vi "Test Different Internal ImageResIDs.vi"(8 "error in (no error)":errorcluster) -> (0 "error out":errorcluster)   [LabVIEW 2026, in "VILab.lvlib"]
uses:
  VILab.lvlib
  SubVIs/Find Resource by Type (String).vi
  CTLs/Resource.ctl
  <vilib>/Utility/traverseref.llb/VI Scripting - Traverse.lvlib
  <vilib>/Utility/traverseref.llb/TRef TravTarget.ctl
panel:
  out "i":i32
  out "Last Error":errorcluster
  out "Working IDs":i32[](array[numeric])
  in  "stop":bool
  # "tried up to -5000"
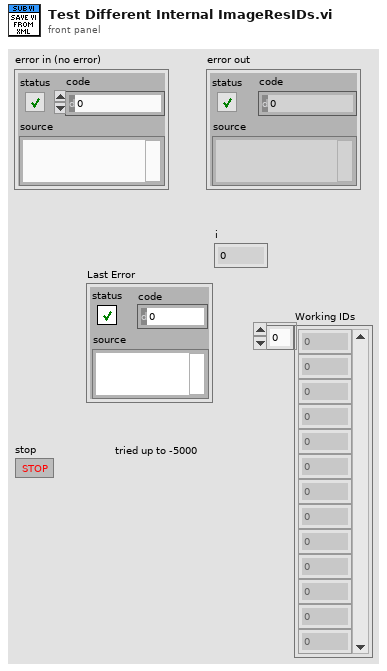
[diagram p1: front panel]
types:
  T1 = typedef "TRef TravTarget.ctl" = enum16{"FP", "BD", "Other"}
  T2 = typedef "VILab.lvlib/Resource.ctl" = cluster{"type":u32, "id":i32, "name":string, "binary data":string}
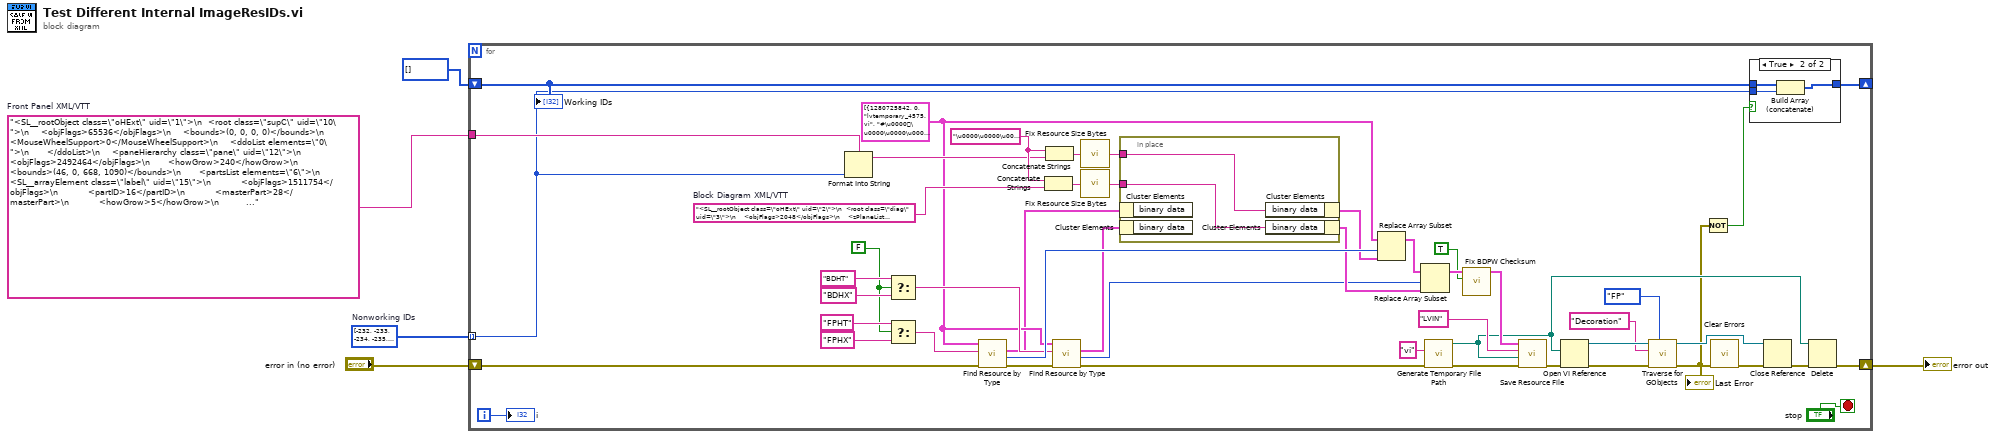
[diagram p0: block diagram]
diagram:
  w1 = i32[] [-232, -233, -234, -235, -236, -237, -367, -368, -369, -370, -371, -372, -392, -501, -502, -503, -504, -532, -542, -642, -643, -646, -647, -765, -770, -784, -785, -840, -841, -842, -843, -844, -845, -846, -847, -848, -849, -850, -851, -852, -853, -854, -855, -856, -857, -858, -859, -860, -861, -862, -863, -864, -865, -866, -867, -868, -869, -870, -871, -872, -873, -874, -875, -876, -877, -878, -879, -880, -881, -882, -883, -884, -885, -886, -887, -888, -889, -890, -891, -892, -893, -894, -895, -896, -897, -898, -899, -900, -901, -902, -903, -904, -905, -906, -907, -908, -909, -910, -911, -912, -913, -914, -915, -916, -917, -918, -919, -920, -921, -922, -923, -924, -925, -926, -927, -928, -929, -930, -931, -932, -933, -934, -935, -936, -937, -938, -939, -940, -941, -942, -943, -944, -945, -946, -947, -948, -949, -950, -951, -952, -953, -954, -955, -956, -957, -958, -959, -960, -961, -962, -963, -964, -965, -966, -967, -968, -969, -970, -971, -972, -973, -974, -975, -976, -977, -978, -979, -980, -981, -982, -983, -984, -985, -986, -987, -988, -989, -990, -991, -992, -993, -994, -995, -996, -997, -998, -999, -1031, -1032, -1033, -1034, -1035, -1036, -1037, -1038, -1039, -1040, -1041, -1042, -1043, -1044, -1045, -1046, -1047, -1048, -1049, -1050, -1051, -1052, -1053, -1054, -1055, -1056, -1057, -1058, -1059, -1060, -1061, -1062, -1063, -1064, -1065, -1066, -1067, -1068, -1069, -1070, -1071, -1072, -1073, -1074, -1075, -1076, -1077, -1078, -1079, -1080, -1081, -1082, -1083, -1084, -1085, -1086, -1087, -1088, -1089, -1090, -1091, -1092, -1093, -1094, -1095, -1096, -1097, -1098, -1099, -1100, -1101, -1102, -1103, -1104, -1105, -1106, -1107, -1108, -1109, -1110, -1111, -1112, -1113, -1114, -1115, -1116, -1117, -1118, -1119, -1120, -1121, -1122, -1123, -1124, -1125, -1126, -1127, -1128, -1129, -1130, -1131, -1132, -1133, -1134, -1135, -1136, -1137, -1138, -1139, -1140, -1141, -1142, -1143, -1144, -1145, -1146, -1147, -1148, -1149, -1150, -1151, -1152, -1153, -1154, -1155, -1156, -1157, -1158, -1159, -1160, -1161, -1162, -1163, -1164, -1165, -1166, -1167, -1168, -1169, -1170, -1171, -1172, -1173, -1174, -1175, -1176, -1177, -1178, -1179, -1180, -1181, -1182, -1183, -1184, -1185, -1186, -1187, -1188, -1189, -1190, -1191, -1192, -1193, -1194, -1195, -1196, -1197, -1198, -1199, -1200, -1201, -1202, -1203, -1204, -1205, -1206, -1207, -1208, -1209, -1210, -1211, -1212, -1213, -1214, -1215, -1216, -1217, -1218, -1219, -1220, -1221, -1222, -1223, -1224, -1225, -1226, -1227, -1228, -1229, -1230, -1231, -1232, -1233, -1234, -1235, -1236, -1237, -1238, -1239, -1240, -1241, -1242, -1243, -1244, -1245, -1246, -1247, -1248, -1249, -1250, -1251, -1252, -1253, -1254, -1255, -1256, -1257, -1258, -1259, -1260, -1261, -1262, -1263, -1264, -1265, -1266, -1267, -1268, -1269, -1270, -1271, -1272, -1273, -1274, -1275, -1276, -1277, -1278, -1279, -1280, -1281, -1282, -1283, -1284, -1285, -1286, -1287, -1288, -1289, -1290, -1291, -1292, -1293, -1294, -1295, -1296, -1297, -1298, -1299, -1300, -1301, -1302, -1303, -1304, -1305, -1306, -1307, -1308, -1309, -1310, -1311, -1312, -1313, -1314, -1315, -1316, -1317, -1318, -1319, -1320, -1321, -1322, -1323, -1324, -1325, -1326, -1327, -1328, -1329, -1330, -1331, -1332, -1333, -1334, -1335, -1336, -1337, -1338, -1339, -1340, -1341, -1342, -1343, -1344, -1345, -1346, -1347, -1348, -1349, -1350, -1351, -1352, -1353, -1354, -1355, -1356, -1357, -1358, -1359, -1360, -1361, -1362, -1363, -1364, -1365, -1366, -1367, -1368, -1369, -1370, -1371, -1372, -1373, -1374, -1375, -1376, -1377, -1378, -1379, -1380, -1381, -1382, -1383, -1384, -1385, -1386, -1387, -1388, -1389, -1390, -1391, -1392, -1393, -1394, -1395, -1396, -1397, -1398, -1399, -1400, -1401, -1402, -1403, -1404, -1405, -1406, -1407, -1408, -1409, -1410, -1411, -1412, -1413, -1414, -1415, -1416, -1417, -1418, -1419, -1420, -1421, -1422, -1423, -1424, -1425, -1426, -1427, -1428, -1429, -1430, -1431, -1432, -1433, -1434, -1435, -1436, -1437, -1438, -1439, -1440, -1441, -1442, -1443, -1444, -1445, -1446, -1447, -1448, -1449, -1450, -1451, -1452, -1453, -1454, -1455, -1456, -1457, -1458, -1459, -1460, -1461, -1462, -1463, -1464, -1465, -1466, -1467, -1468, -1469, -1470, -1471, -1472, -1473, -1474, -1475, -1476, -1477, -1478, -1479, -1480, -1481, -1482, -1483, -1484, -1485, -1486, -1487, -1488, -1489, -1490, -1491, -1492, -1493, -1494, -1495, -1496, -1497, -1498, -1499, -1500, -1501, -1502, -1503, -1504, -1505, -1506, -1507, -1508, -1509, -1510, -1511, -1512, -1513, -1514, -1515, -1516, -1517, -1518, -1519, -1520, -1521, -1522, -1523, -1524, -1525, -1526, -1527, -1528, -1529, -1530, -1531, -1532, -1533, -1534, -1535, -1536, -1537, -1538, -1539, -1540, -1541, -1542, -1543, -1544, -1545, -1546, -1547, -1548, -1549, -1550, -1551, -1552, -1553, -1554, -1555, -1556, -1557, -1558, -1559, -1560, -1561, -1562, -1563, -1564, -1565, -1566, -1567, -1568, -1569, -1570, -1571, -1572, -1573, -1574, -1575, -1576, -1577, -1578, -1579, -1580, -1581, -1582, -1583, -1584, -1585, -1586, -1587, -1588, -1589, -1590, -1591, -1592, -1593, -1594, -1595, -1596, -1597, -1598, -1599, -1600, -1601, -1602, -1603, -1604, -1605, -1606, -1607, -1608, -1609, -1610, -1611, -1612, -1613, -1614, -1615, -1616, -1617, -1618, -1619, -1620, -1621, -1622, -1623, -1624, -1625, -1626, -1627, -1628, -1629, -1630, -1631, -1632, -1633, -1634, -1635, -1636, -1637, -1638, -1639, -1640, -1641, -1642, -1643, -1644, -1645, -1646, -1647, -1648, -1649, -1650, -1651, -1652, -1653, -1654, -1655, -1656, -1657, -1658, -1659, -1660, -1661, -1662, -1663, -1664, -1665, -1666, -1667, -1668, -1669, -1670, -1671, -1672, -1673, -1674, -1675, -1676, -1677, -1678, -1679, -1680, -1681, -1682, -1683, -1684, -1685, -1686, -1687, -1688, -1689, -1690, -1691, -1692, -1693, -1694, -1695, -1696, -1697, -1698, -1699, -1700, -1701, -1702, -1703, -1704, -1705, -1706, -1707, -1708, -1709, -1710, -1711, -1712, -1713, -1714, -1715, -1716, -1717, -1718, -1719, -1720, -1721, -1722, -1723, -1724, -1725, -1726, -1727, -1728, -1729, -1730, -1731, -1732, -1733, -1734, -1735, -1736, -1737, -1738, -1739, -1740, -1741, -1742, -1743, -1744, -1745, -1746, -1747, -1748, -1749, -1750, -1751, -1752, -1753, -1754, -1755, -1756, -1757, -1758, -1759, -1760, -1761, -1762, -1763, -1764, -1765, -1766, -1767, -1768, -1769, -1770, -1771, -1772, -1773, -1774, -1775, -1776, -1777, -1778, -1779, -1780, -1781, -1782, -1783, -1784, -1785, -1786, -1787, -1788, -1789, -1790, -1791, -1792, -1793, -1794, -1795, -1796, -1797, -1798, -1799, -1800, -1801, -1802, -1803, -1804, -1805, -1806, -1807, -1808, -1809, -1810, -1811, -1812, -1813, -1814, -1815, -1816, -1817, -1818, -1819, -1820, -1821, -1822, -1823, -1824, -1825, -1826, -1827, -1828, -1829, -1830, -1831, -1832, -1833, -1834, -1835, -1836, -1837, -1838, -1839, -1840, -1841, -1842, -1843, -1844, -1845, -1846, -1847, -1848, -1849, -1850, -1851, -1852, -1853, -1854, -1855, -1856, -1857, -1858, -1859, -1860, -1861, -1862, -1863, -1864, -1865, -1866, -1867, -1868, -1869, -1870, -1871, -1872, -1873, -1874, -1875, -1876, -1877, -1878, -1879, -1880, -1881, -1882, -1883, -1884, -1885, -1886, -1887, -1888, -1889, -1890, -1891, -1892, -1893, -1894, -1895, -1896, -1897, -1898, -1899, -1900, -1901, -1902, -1903, -1904, -1905, -1906, -1907, -1908, -1909, -1910, -1911, -1912, -1913, -1914, -1915, -1916, -1917, -1918, -1919, -1920, -1921, -1922, -1923, -1924, -1925, -1926, -1927, -1928, -1929, -1930, -1931, -1932, -1933, -1934, -1935, -1936, -1937, -1938, -1939, -1940, -1941, -1942, -1943, -1944, -1945, -1946, -1947, -1948, -1949, -1950, -1951, -1952, -1953, -1954, -1955, -1956, -1957, -1958, -1959, -1960, -1961, -1962, -1963, -1964, -1965, -1966, -1967, -1968, -1969, -1970, -1971, -1972, -1973, -1974, -1975, -1976, -1977, -1978, -1979, -1980, -1981, -1982, -1983, -1984, -1985, -1986, -1987, -1988, -1989, -1990, -1991, -1992, -1993, -1994, -1995, -1996, -1997, -1998, -1999, -2110, -2111, -2112, -2113, -2114, -2115, -2116, -2117, -2118, -2119, -2120, -2121, -2122, -2123, -2124, -2125, -2126, -2127, -2128, -2129, -2130, -2131, -2132, -2133, -2134, -2135, -2136, -2137, -2138, -2139, -2140, -2141, -2142, -2143, -2144, -2145, -2146, -2147, -2148, -2149, -2150, -2151, -2152, -2153, -2154, -2155, -2156, -2157, -2158, -2159, -2160, -2161, -2162, -2163, -2164, -2165, -2166, -2167, -2168, -2169, -2170, -2171, -2172, -2173, -2174, -2175, -2176, -2177, -2178, -2179, -2180, -2181, -2182, -2183, -2184, -2185, -2186, -2187, -2188, -2189, -2190, -2191, -2192, -2193, -2194, -2195, -2196, -2197, -2198, -2199, -2200, -2201, -2202, -2203, -2204, -2205, -2206, -2207, -2208, -2209, -2210, -2211, -2212, -2213, -2214, -2215, -2216, -2217, -2218, -2219, -2220, -2221, -2222, -2223, -2224, -2225, -2226, -2227, -2228, -2229, -2230, -2231, -2232, -2233, -2234, -2235, -2236, -2237, -2238, -2239, -2240, -2241, -2242, -2243, -2244, -2245, -2246, -2247, -2248, -2249, -2250, -2251, -2252, -2253, -2254, -2255, -2256, -2257, -2258, -2259, -2260, -2261, -2262, -2263, -2264, -2265, -2266, -2267, -2268, -2269, -2270, -2271, -2272, -2273, -2274, -2275, -2276, -2277, -2278, -2279, -2280, -2281, -2282, -2283, -2284, -2285, -2286, -2287, -2288, -2289, -2290, -2291, -2292, -2293, -2294, -2295, -2296, -2297, -2298, -2299, -2300, -2301, -2302, -2303, -2304, -2305, -2306, -2307, -2308, -2309, -2310, -2311, -2312, -2313, -2314, -2315, -2316, -2317, -2318, -2319, -2320, -2321, -2322, -2323, -2324, -2325, -2326, -2327, -2328, -2329, -2330, -2331, -2332, -2333, -2334, -2335, -2336, -2337, -2338, -2339, -2340, -2341, -2342, -2343, -2344, -2345, -2346, -2347, -2348, -2349, -2350, -2351, -2352, -2353, -2354, -2355, -2356, -2357, -2358, -2359, -2360, -2361, -2362, -2363, -2364, -2365, -2366, -2367, -2368, -2369, -2370, -2371, -2372, -2373, -2374, -2375, -2376, -2377, -2378, -2379, -2380, -2381, -2382, -2383, -2384, -2385, -2386, -2387, -2388, -2389, -2390, -2391, -2392, -2393, -2394, -2395, -2396, -2397, -2398, -2399, -2400, -2401, -2402, -2403, -2404, -2405, -2406, -2407, -2408, -2409, -2410, -2411, -2412, -2413, -2414, -2415, -2416, -2417, -2418, -2419, -2420, -2421, -2422, -2423, -2424, -2425, -2426, -2427, -2428, -2429, -2430, -2431, -2432, -2433, -2434, -2435, -2436, -2437, -2438, -2439, -2440, -2441, -2442, -2443, -2444, -2445, -2446, -2447, -2448, -2449, -2450, -2451, -2452, -2453, -2454, -2455, -2456, -2457, -2458, -2459, -2460, -2461, -2462, -2463, -2464, -2465, -2466, -2467, -2468, -2469, -2470, -2471, -2472, -2473, -2474, -2475, -2476, -2477, -2478, -2479, -2480, -2481, -2482, -2483, -2484, -2485, -2486, -2487, -2488, -2489, -2490, -2491, -2492, -2493, -2494, -2495, -2496, -2497, -2498, -2499, -2500, -2501, -2502, -2503, -2504, -2505, -2506, -2507, -2508, -2509, -2510, -2511, -2512, -2513, -2514, -2515, -2516, -2517, -2518, -2519, -2520, -2521, -2522, -2523, -2524, -2525, -2526, -2527, -2528, -2529, -2530, -2531, -2532, -2533, -2534, -2535, -2536, -2537, -2538, -2539, -2540, -2541, -2542, -2543, -2544, -2545, -2546, -2547, -2548, -2549, -2550, -2551, -2552, -2553, -2554, -2555, -2556, -2557, -2558, -2559, -2560, -2561, -2562, -2563, -2564, -2565, -2566, -2567, -2568, -2569, -2570, -2571, -2572, -2573, -2574, -2575, -2576, -2577, -2578, -2579, -2580, -2581, -2582, -2583, -2584, -2585, -2586, -2587, -2588, -2589, -2590, -2591, -2592, -2593, -2594, -2595, -2596, -2597, -2598, -2599, -2600, -2601, -2602, -2603, -2604, -2605, -2606, -2607, -2608, -2609, -2610, -2611, -2612, -2613, -2614, -2615, -2616, -2617, -2618, -2619, -2620, -2621, -2622, -2623, -2624, -2625, -2626, -2627, -2628, -2629, -2630, -2631, -2632, -2633, -2634, -2635, -2636, -2637, -2638, -2639, -2640, -2641, -2642, -2643, -2644, -2645, -2646, -2647, -2648, -2649, -2650, -2651, -2652, -2653, -2654, -2655, -2656, -2657, -2658, -2659, -2660, -2661, -2662, -2663, -2664, -2665, -2666, -2667, -2668, -2669, -2670, -2671, -2672, -2673, -2674, -2675, -2676, -2677, -2678, -2679, -2680, -2681, -2682, -2683, -2684, -2685, -2686, -2687, -2688, -2689, -2690, -2691, -2692, -2693, -2694, -2695, -2696, -2697, -2698, -2699, -2700, -2701, -2702, -2703, -2704, -2705, -2706, -2707, -2708, -2709, -2710, -2711, -2712, -2713, -2714, -2715, -2716, -2717, -2718, -2719, -2720, -2721, -2722, -2723, -2724, -2725, -2726, -2727, -2728, -2729, -2730, -2731, -2732, -2733, -2734, -2735, -2736, -2737, -2738, -2739, -2740, -2741, -2742, -2743, -2744, -2745, -2746, -2747, -2748, -2749, -2750, -2751, -2752, -2753, -2754, -2755, -2756, -2757, -2758, -2759, -2760, -2761, -2762, -2763, -2764, -2765, -2766, -2767, -2768, -2769, -2770, -2771, -2772, -2773, -2774, -2775, -2776, -2777, -2778, -2779, -2780, -2781, -2782, -2783, -2784, -2785, -2786, -2787, -2788, -2789, -2790, -2791, -2792, -2793, -2794, -2795, -2796, -2797, -2798, -2799, -2800, -2801, -2802, -2803, -2804, -2805, -2806, -2807, -2808, -2809, -2810, -2811, -2812, -2813, -2814, -2815, -2816, -2817, -2818, -2819, -2820, -2821, -2822, -2823, -2824, -2825, -2826, -2827, -2828, -2829, -2830, -2831, -2832, -2833, -2834, -2835, -2836, -2837, -2838, -2839, -2840, -2841, -2842, -2843, -2844, -2845, -2846, -2847, -2848, -2849, -2850, -2851, -2852, -2853, -2854, -2855, -2856, -2857, -2858, -2859, -2860, -2861, -2862, -2863, -2864, -2865, -2866, -2867, -2868, -2869, -2870, -2871, -2872, -2873, -2874, -2875, -2876, -2877, -2878, -2879, -2880, -2881, -2882, -2883, -2884, -2885, -2886, -2887, -2888, -2889, -2890, -2891, -2892, -2893, -2894, -2895, -2896, -2897, -2898, -2899, -2900, -2901, -2902, -2903, -2904, -2905, -2906, -2907, -2908, -2909, -2910, -2911, -2912, -2913, -2914, -2915, -2916, -2917, -2918, -2919, -2920, -2921, -2922, -2923, -2924, -2925, -2926, -2927, -2928, -2929, -2930, -2931, -2932, -2933, -2934, -2935, -2936, -2937, -2938, -2939, -2940, -2941, -2942, -2943, -2944, -2945, -2946, -2947, -2948, -2949, -2950, -2951, -2952, -2953, -2954, -2955, -2956, -2957, -2958, -2959, -2960, -2961, -2962, -2963, -2964, -2965, -2966, -2967, -2968, -2969, -2970, -2971, -2972, -2973, -2974, -2975, -2976, -2977, -2978, -2979, -2980, -2981, -2982, -2983, -2984, -2985, -2986, -2987, -2988, -2989, -2990, -2991, -2992, -2993, -2994, -2995, -2996, -2997, -2998, -2999]  # Nonworking IDs
  w3 = "<SL__rootObject class=\"oHExt\" uid=\"1\">\n  <root class=\"supC\" uid=\"10\">\n    <objFlags>65536</objFlags>\n    <bounds>(0, 0, 0, 0)</bounds>\n    <MouseWheelSupport>0</MouseWheelSupport>\n    <ddoList elements=\"0\">\n      </ddoList>\n    <paneHierarchy class=\"pane\" uid=\"12\">\n      <objFlags>2492464</objFlags>\n      <howGrow>240</howGrow>\n      <bounds>(46, 0, 668, 1090)</bounds>\n      <partsList elements=\"6\">\n        <SL__arrayElement class=\"label\" uid=\"15\">\n          <objFlags>1511754</objFlags>\n          <partID>16</partID>\n          <masterPart>28</masterPart>\n          <howGrow>5</howGrow>\n          <bounds>(0, 0, 17, 29)</bounds>\n          <image class=\"Image\">\n            <ImageResID>-9</ImageResID>\n            </image>\n          <fgColor>01000000</fgColor>\n          <bgColor>01000000</bgColor>\n          <textRec class=\"textHair\">\n            <mode>1028</mode>\n            <text>\"Pane\"</text>\n            <bgColor>01000000</bgColor>\n            </textRec>\n          </SL__arrayElement>\n        <SL__arrayElement class=\"cosm\" uid=\"16\">\n          <objFlags>3442</objFlags>\n          <partID>39</partID>\n          <masterPart>28</masterPart>\n          <howGrow>194</howGrow>\n          <bounds>(0, 1073, 605, 1090)</bounds>\n          <image class=\"Image\">\n            <ImageResID>0</ImageResID>\n            </image>\n          <bgColor>00B3B3B3</bgColor>\n          </SL__arrayElement>\n        <SL__arrayElement class=\"cosm\" uid=\"17\">\n          <objFlags>3442</objFlags>\n          <partID>38</partID>\n          <masterPart>28</masterPart>\n          <howGrow>56</howGrow>\n          <bounds>(605, 0, 622, 1073)</bounds>\n          <image class=\"Image\">\n            <ImageResID>0</ImageResID>\n            </image>\n          <bgColor>00B3B3B3</bgColor>\n          </SL__arrayElement>\n        <SL__arrayElement class=\"cosm\" uid=\"18\">\n          <objFlags>7539</objFlags>\n          <partID>44</partID>\n          <masterPart>28</masterPart>\n          <howGrow>10</howGrow>\n          <bounds>(605, 1073, 622, 1090)</bounds>\n          <image class=\"Image\">\n            <ImageResID>-365</ImageResID>\n            </image>\n          <fgColor>00B3B3B3</fgColor>\n          <bgColor>00B3B3B3</bgColor>\n          </SL__arrayElement>\n        <SL__arrayElement class=\"cosm\" uid=\"19\">\n          <objFlags>4211</objFlags>\n          <partID>28</partID>\n          <howGrow>120</howGrow>\n          <bounds>(0, 0, 605, 1073)</bounds>\n          <image class=\"Image\">\n            <ImageResID>-704</ImageResID>\n            </image>\n          <fgColor>00E2E2E2</fgColor>\n          <bgColor>00E2E2E2</bgColor>\n          </SL__arrayElement>\n        <SL__arrayElement class=\"annex\" uid=\"20\">\n          <partID>66</partID>\n          </SL__arrayElement>\n        </partsList>\n      <paneFlags>331089</paneFlags>\n      <minPaneSize>(1,1)</minPaneSize>\n      <docBounds>(-79, -136, 605, 1073)</docBounds>\n      <zPlaneList elements=\"1\">\n        <SL__arrayElement class=\"cosm\" uid=\"78\">\n          <objFlags>1</objFlags>\n          <bounds>(26, 132, 63, 169)</bounds>\n          <image class=\"Image\">\n            <ImageResID>%d</ImageResID>\n            <ImageInternalsResID>2</ImageInternalsResID>\n            </image>\n          </SL__arrayElement>\n        </zPlaneList>\n      <image class=\"Image\">\n        <ImageResID>0</ImageResID>\n        </image>\n      </paneHierarchy>\n    <savedSize>(0, 0, 0, 0)</savedSize>\n    <conPane class=\"conPane\" uid=\"21\">\n      <conId>4815</conId>\n      <cons elements=\"12\">\n        </cons>\n      </conPane>\n    <keyMappingList class=\"keyMapList\" uid=\"22\">\n      </keyMappingList>\n    </root>\n  <pBounds>(46, 0, 668, 1090)</pBounds>\n  <dBounds>(0, 0, 0, 0)</dBounds>\n  <origin>(576,261)</origin>\n  <instrStyle>31</instrStyle>\n  <blinkList elements=\"0\">\n    </blinkList>\n  </SL__rootObject>"  # Front Panel XML/VTT
  n1 = for {
    shift-right: [w17] -> w4
    shift-left: "error in (no error)" -> [w31]
    tunnel: w3 -> [w27]
    shift-right: [w24] -> _
    shift-left: i32[] [] -> [w25]
    tunnel: w1 -> [w11] mode=indexing
    i -> [w9]
    stop <- "stop" stop-if-true
    w8 = T2[] [{"type"=1280725842, "id"=0, "name"="lvtemporary_4575.vi", "binary data"="#\u0000\u0000\u0000\u0000\u0000\u0000 \u0000\u0006\u0000\u0000\u0000\u0000\u0004\u0000\u0003\u0000<\u0000\u0000\u0000\u001f@\u0002\u0000\u0000\u0000\u0000\u0001\u0000\u0001\u0000\u0002ÿÿÿÿ\u0000\u0000\u0000\u0000\u0000\u0000\u0000\u0000\u0000\u0000\u0000\u0000\u0000\u0000\u0000\u0000\u0000\u0000\u0000\u0000\u0000\u0000\u0000\u0000\u0000\u0000\u0000\u0000\u0000\u0000\u0000\f\u0000\u0000\u0000\u0010\u0000\u0000\u0000\u0000\u0000\u0000\u0000\u0000\u0000\u0000\u0000\u0000\u0000\u0000\u0000\u0000\u0000\u0000\u0000\u0000Ô\u001dÙ\u0000²\u0004é\tìøB~\u0000\u0000\u0000\u0000\u0000\u0000\u0000\u0000\u0000\u0000\u0000\u0000\u0000\u0000\u0000\u0000\u0000\u0000\u0000\u0000\u0000\u0000\u0000\u0000\u0001\u0000\u0000\u0000ÿÿÿÿÔ\u001dÙ\u0000²\u0004é\tìøB~"}, {"type"=1381258055, "id"=0, "name"="", "binary data"="\u0000\u0000\u0000\u0000\u0000\u0000\u0000\u0000\u0000\u0000\u0000\u0000\u0000\u0000\u0000\u0000"}, {"type"=1986359923, "id"=4, "name"="", "binary data"="#6€\u0006\u0000\u0000\u000623.3.6\u0000"}, {"type"=1129270864, "id"=0, "name"="", "binary data"="\u0000\u0001"}, {"type"=1279882857, "id"=0, "name"="", "binary data"="\u0000\u0001LVIN\u0000\u0000\u0000\u0000\u0000\u0003"}, {"type"=1111773271, "id"=0, "name"="", "binary data"="Ô\u001dÙ\u0000²\u0004é\tìøB~K@I.b\u0001-\u001amå­U\u0006òó½KSû÷¸J@\u001cD­)T¬\u0012"}, {"type"=1229147982, "id"=0, "name"="", "binary data"="ÿÿÿÿ\u0000\u0000\u0001\u0000\u0000\u0001ÿü\u0001\u0000T\u0001ÿT\u0001ûT\u0001u\u0004\u0001u$\u0001®T\u0001®T\u0001ß$\u0001ÿ\u0004\u0001\u0000\u001c\u0001\u0000\u0016\u0001\u0010ñ;\u0012a$\u0017\u001dÿòaIñ2\u0016\u0001\u0018\u0001x\u0000\u0001\u0000\u0000\u0001\u0000\u0000\u0001\u0000\u0000\u0001\u0000\u0000\u0001\u0000\u0000\u0001\u0000\u0000\u0001\u0000\u0000\u0001\u0000\u0000\u0001ÿÿÿÿ"}, {"type"=1768123448, "id"=0, "name"="", "binary data"="ÿÿÿÿÿÿÿÿÿÿÿÿÿÿÿÿÿÿÿÿÿÿÿÿÿÿÿÿÿÿÿÿÿ\u0000\u0000\u0000\u0000\u0000\u0000\u0000\u0000\u0000\u0000\u0000\u0000\u0000\u0000\u0000\u0000\u0000\u0000\u0000\u0000\u0000\u0000\u0000\u0000\u0000\u0000\u0000\u0000\u0000\u0000ÿÿ\u0000\u0000\u0000\u0000\u0000\u0000\u0000\u0000\u0000\u0000\u0000\u0000\u0000\u0000\u0000\u0000\u0000\u0000\u0000\u0000\u0000\u0000\u0000\u0000\u0000\u0000\u0000\u0000\u0000\u0000ÿÿ\u0000\u0000ÿÿÿÿÿÿÿÿÿÿÿÿÿÿÿÿÿÿÿ\u0000\u0000\u0000\u0000\u0000\u0000\u0000\u0000\u0000ÿÿ\u0000\u0000ÿùùùùùùùùùùùù÷ù,ù,à\u0000\u0000\u0000\u0000\u0000\u0000\u0000\u0000\u0000ÿÿ\u0000\u0000ÿùÿÿÿÿÿÿÿÿÿÿÿ÷ù,ù,ÿ\u0000\u0000\u0000\u0000\u0000\u0000\u0000\u0000\u0000ÿÿ\u0000\u0000ÿùÿèäèÿÿÿèäèÿ÷ü+ü,ÿ\u0000\u0000\u0000\u0000\u0000\u0000\u0000\u0000\u0000ÿÿ\u0000\u0000ÿùÿäÿäÿÿÿäÿäÿ÷,,,,à\u0000\u0000\u0000\u0000\u0000\u0000\u0000\u0000\u0000ÿÿ\u0000\u0000ÿùèäÿäèÿèäÿäè÷+ü+,ÿ\u0000\u0000\u0000\u0000\u0000\u0000\u0000\u0000\u0000ÿÿ\u0000\u0000ÿùäèÿèäÿäèÿèä÷ü\bü,ÿ\u0000\u0000\u0000\u0000\u0000\u0000\u0000\u0000\u0000ÿÿ\u0000\u0000ÿùäÿÿÿäÿäÿÿÿä÷ü\bü,ÿ\u0000\u0000\u0000\u0000\u0000\u0000\u0000\u0000\u0000ÿÿ\u0000\u0000ÿùÿÿÿÿèäèÿÿÿÿ÷+ü+,ÿ\u0000\u0000\u0000\u0000\u0000\u0000\u0000\u0000\u0000ÿÿ\u0000\u0000ÿùÿÿÿÿÿÿÿÿÿÿÿ÷,,,,ÿ\u0000\u0000\u0000\u0000\u0000\u0000\u0000\u0000\u0000ÿÿ\u0000\u0000ÿ÷÷÷÷÷÷÷÷÷÷÷÷÷,,ƒƒÿ\u0000\u0000\u0000\u0000\u0000\u0000\u0000\u0000\u0000ÿÿ\u0000\u0000ÿ,,,,,,,,,,,,,,,ƒ\u0005ƒƒ\u0000\u0000\u0000\u0000\u0000\u0000\u0000\u0000ÿÿ\u0000\u0000ÿ,ü,,,,,ü,,,,###ƒ\u0005\u0005\u0005ƒƒ\u0000\u0000\u0000\u0000\u0000\u0000ÿÿ\u0000\u0000ÿüðü,,,ü#ü,##,,,ƒ\u0005\u0005ÿ\u0005\u0005ƒƒ\u0000\u0000\u0000\u0000ÿÿ\u0000\u0000ÿ,ï,,,,#,,#,,,,,ƒ\u0005ÿÿÿ\u0005\u0005\u0005ƒ##\u0000ÿÿ\u0000\u0000ÿÿðÿÿÿ#ÿÿ#ÿÿÿÿÿÿƒ\u0005\u0005ÿ\u0005..."}, {"type"=1414091852, "id"=0, "name"="", "binary data"="\tSource VI"}, {"type"=1129333554, "id"=0, "name"="", "binary data"="\u0000\u0001"}, {"type"=1279878768, "id"=0, "name"="", "binary data"="\u0000\u0001FPHP\u0000\u0000\u0000\u0000\u0000\u0003"}, {"type"=1179665784, "id"=0, "name"="", "binary data"="\u0000\u0000\u0000\u0000"}, {"type"=1346978627, "id"=2, "name"="", "binary data"="\u0000\u0002\u0000\u0001\u0000H\u0000„\u0000l\u0000¨"}, {"type"=1179666520, "id"=0, "name"="", "binary data"="\u0000\u0000\u000eÆ<SL__rootObject class=\"oHExt\" uid=\"1\">\n  <root class=\"supC\" uid=\"10\">\n    <objFlags>65536</objFlags>\n    <bounds>(0, 0, 0, 0)</bounds>\n    <MouseWheelSupport>0</MouseWheelSupport>\n    <ddoList elements=\"0\">\n      </ddoList>\n    <paneHierarchy class=\"pane\" uid=\"12\">\n      <objFlags>2492464</objFlags>\n      <howGrow>240</howGrow>\n      <bounds>(46, 0, 668, 1090)</bounds>\n      <partsList elements=\"6\">\n        <SL__arrayElement class=\"label\" uid=\"15\">\n          <objFlags>1511754</objFlags>\n          <partID>16</partID>\n          <masterPart>28</masterPart>\n          <howGrow>5</howGrow>\n          <bounds>(0, 0, 17, 29)</bounds>\n          <image class=\"Image\">\n            <ImageResID>-9</ImageResID>\n            </image>\n          <fgColor>01000000</fgColor>\n          <bgColor>01000000</bgColor>\n          <textRec class=\"textHair\">\n            <mode>1028</mode>\n            <text>\"Pane\"</text>\n            <bgColor>01000000</bgColor>\n            </textRec>\n          </SL__arrayElement>\n        <SL__arrayElement class=\"cosm\" uid=\"16\">\n          <objFlags>3442</objFlags>\n          <partID>39</partID>\n          <masterPart>28</masterPart>\n          <howGrow>194</howGrow>\n          <bounds>(0, 1073, 605, 1090)</bounds>\n          <image class=\"Image\">\n            <ImageResID>0</ImageResID>\n            </image>\n          <bgColor>00B3B3B3</bgColor>\n          </SL__arrayElement>\n        <SL__arrayElement class=\"cosm\" uid=\"17\">\n          <objFlags>3442</objFlags>\n          <partID>38</partID>\n          <masterPart>28</masterPart>\n          <howGrow>56</howGrow>\n          <bounds>(605, 0, 622, 1073)</bounds>\n          <image class=\"Image\">\n            <ImageResID>0</ImageResID>\n            </image>\n          <bgColor>00B3B3B3</bgColor>\n          </SL__arrayElement>\n        <SL__arrayElement class=\"cosm\" uid=\"18\">\n          <objFlags>7539</objFlags>\n          <partID>44</partID>\n          <masterPart>28</masterPart>\n          <howGrow>10</howGrow>\n          <bounds>(605, 1073, 622, 1090)</bounds>\n          <image class=\"Image\">\n            <ImageResID>-365</ImageResID>\n            </image>\n          <fgColor>00B3B3B3</fgColor>\n          <bgColor>00B3B3B3</bgColor>\n          </SL__arrayElement>\n        <SL__arrayElement class=\"cosm\" uid=\"19\">\n          <objFlags>4211</objFlags>\n          <partID>28</partID>\n          <howGrow>120</howGrow>\n          <bounds>(0, 0, 605, 1073)</bounds>\n          <image class=\"Image\">\n            <ImageResID>-704</ImageResID>\n            </image>\n          <fgColor>00E2E2E2</fgColor>\n          <bgColor>00E2E2E2</bgColor>\n          </SL__arrayElement>\n        <SL__arrayElement class=\"annex\" uid=\"20\">\n          <partID>66</partID>\n          </SL__arrayElement>\n        </partsList>\n      <paneFlags>331089</paneFlags>\n      <minPaneSize>(1,1)</minPaneSize>\n      <docBounds>(-79, -136, 605, 1073)</docBounds>\n      <zPlaneList elements=\"1\">\n        <SL__arrayElement class=\"cosm\" uid=\"78\">\n          <objFlags>1</objFlags>\n          <bounds>(26, 132, 63, 169)</bounds>\n          <image class=\"Image\">\n            <ImageResID>-233</ImageResID>\n            <ImageInternalsResID>2</ImageInternalsResID>\n            </image>\n          </SL__arrayElement>\n        </zPlaneList>\n      <image class=\"Image\">\n        <ImageResID>0</ImageResID>\n        </image>\n      </paneHierarchy>\n    <savedSize>(0, 0, 0, 0)</savedSize>\n    <conPane class=\"conPane\" uid=\"21\">\n      <conId>4815</conId>\n      <cons elements=\"12\">\n        </cons>\n      </conPane>\n    <keyMappingList class=\"keyMapList\" uid=\"22\">\n      </keyMappingList>\n    </root>\n  <pBounds>(46, 0, 668, 1090)</pBounds>\n  <dBounds>(0, 0, 0, 0)</dBounds>\n  <origin>(576,261)</origin>\n  <instrStyle>31</instrStyle>\n  <blinkList elements=\"0\">\n    </blinkList>\n  </SL__rootObject>\n"}, {"type"=1179669317, "id"=0, "name"="", "binary data"="\u0000\u0000\u0000\u0010"}, {"type"=1448100944, "id"=0, "name"="", "binary data"="\u0000\u0000\u0000\u0000"}, {"type"=1279877732, "id"=0, "name"="", "binary data"="\u0000\u0001BDHP\u0000\u0000\u0000\u0000\u0000\u0003"}, {"type"=1111770488, "id"=0, "name"="", "binary data"="\u0000\u0000\u0000\u0000"}, {"type"=1111771224, "id"=0, "name"="", "binary data"="\u0000\u0000\u0002Ï<SL__rootObject class=\"oHExt\" uid=\"2\">\n  <root class=\"diag\" uid=\"3\">\n    <objFlags>2048</objFlags>\n    <zPlaneList elements=\"0\">\n      </zPlaneList>\n    <nodeList elements=\"1\">\n      <SL__arrayElement class=\"sRN\" uid=\"7\">\n        <termList elements=\"0\">\n          </termList>\n        <bounds>(0, 0, 0, 0)</bounds>\n        <shortCount>1</shortCount>\n        <clumpNum>131075</clumpNum>\n        </SL__arrayElement>\n      </nodeList>\n    <signalList elements=\"0\">\n      </signalList>\n    <bgColor>00FFFFFF</bgColor>\n    <firstNodeIdx>1</firstNodeIdx>\n    </root>\n  <pBounds>(46, 0, 651, 1073)</pBounds>\n  <dBounds>(46, 0, 651, 1073)</dBounds>\n  <origin>(625,291)</origin>\n  <instrStyle>31</instrStyle>\n  </SL__rootObject>\n"}, {"type"=1111774021, "id"=0, "name"="", "binary data"="\u0000\u0000\u0000\u0007"}, {"type"=1447646291, "id"=0, "name"="", "binary data"="\u0000\u0000\u0000\u0001\u0000\u0000\u0000\u0014NI.LV.All.SourceOnly\u0000\u0000\u0000\u0015#\u0000€\u0000\u0000\u0000\u0000\u0001\u0000\u0004\u0000!\u0000\u0001\u0000\u0000\u0001\u0000\u0000\u0000\u0000"}, {"type"=1146374224, "id"=0, "name"="", "binary data"="\u0000\u0000"}, {"type"=1297434948, "id"=0, "name"="", "binary data"="\u0000\u0000\u0000N"}, {"type"=1212765012, "id"=0, "name"="", "binary data"="\u0000\u0000\u0000\u0002\u0000\u0000\u0004\u0000\u0000\u0000\u0000\u0007\u0000\u0000\u0000\u0000\u0000\u0000\u0000\u0000\u0000\u0000\u0000\u0000\u0000\u0000\u0000\u0000\u0000\u0000\u0000\u0000\u0000\u0000\u0000\u0000\u0000\u0000\u0000\u0000"}, {"type"=1447253072, "id"=0, "name"="", "binary data"="\u0000\u0000\u0000`xœc```b`a``\baøÀÀÃ€\u001bTà‘Ã\u0005\u0018\u0019\u0018\u0001Œr\u0001Ñ"}, {"type"=1179926850, "id"=128, "name"="", "binary data"="\u0000\u0001\u0000\u0002\u0000\u0003\u0000\u0004\u0000\u0000\u0000H\u0000\u000f\u0004\u0000\u0000\u0000\u0000\u000f\u0000Ù\u0000Ô\u0000\u0000\u0000Q\u0000\u000f\u0004\u0000\u0000\u0000\u0000\u000f\u0000Ù\u0000Ô\u0000\u0000\u0000Z\u0000\u000f\u0004\u0000\u0000\u0000\u0000\u000f\u0000Ù\u0000Ô\u0000\u0000\u0000c€\u0000„\u0000€\u0000\u0000\u000f\u0000Ù\u0000Ô\bSegoe UI\bSegoe UI\bSegoe UI\u00010"}] ("Resources")
    w29 = FALSE ("Use VTT?")
    w28 = "<SL__rootObject class=\"oHExt\" uid=\"2\">\n  <root class=\"diag\" uid=\"3\">\n    <objFlags>2048</objFlags>\n    <zPlaneList elements=\"0\">\n      </zPlaneList>\n    <nodeList elements=\"1\">\n      <SL__arrayElement class=\"sRN\" uid=\"7\">\n        <termList elements=\"0\">\n          </termList>\n        <bounds>(0, 0, 0, 0)</bounds>\n        <shortCount>1</shortCount>\n        <clumpNum>131075</clumpNum>\n        </SL__arrayElement>\n      </nodeList>\n    <signalList elements=\"0\">\n      </signalList>\n    <bgColor>00FFFFFF</bgColor>\n    <firstNodeIdx>1</firstNodeIdx>\n    </root>\n  <pBounds>(46, 0, 651, 1073)</pBounds>\n  <dBounds>(46, 0, 651, 1073)</dBounds>\n  <origin>(625,291)</origin>\n  <instrStyle>31</instrStyle>\n  </SL__rootObject>\n"  # Block Diagram XML/VTT
    w54 = "\u0000\u0000\u0000\u0000"
    n2 = Format Into String(format string=w27, w11) -> (resulting string=w26:string)  [unwired: 2 in, 1 out]
    n3 = Select(t="BDHT", s=w29, f="BDHX") -> (s? t:f=w30:string)
    n4 = Select(t="FPHT", s=w29, f="FPHX") -> (s? t:f=w35:string)
    n5 = call-poly "Find Resource by Type.vi"("error in (no error)"=w31, "Resource Type"=w35, "Resources"=w8) -> ("error out"=w32:errorcluster, "Index"=w49:i32, "Resource"=w7:T2)  [unwired: 4 in, 2 out]
    n6 = Concatenate Strings(w54, w28) -> (w52:string)
    n7 = Concatenate Strings(w54, w26) -> (w53:string)
    n8 = call-poly "Find Resource by Type.vi"("error in (no error)"=w32, "Resource Type"=w30, "Resources"=w8) -> ("error out"=w33:errorcluster, "Index"=w46:i32, "Resource"=w6:T2)  [unwired: 4 in, 2 out]
    n9 = call "Fix Resource Size Bytes.vi"("Data in"=w53) -> ("Data out"=w51:string)
    n10 = call "Fix Resource Size Bytes.vi"("Data in"=w52) -> ("Data out"=w50:string)
    n11 = in-place {
      in-place-border: w51 -> [w60]
      in-place-border: w50 -> [w59]
      n12 = in-place-cluster #1(w7) -> ()  [unwired: 1 out]
      n13 = in-place-cluster #2(w6) -> ()  [unwired: 1 out]
      n14 = in-place-cluster #1("binary data"=w60) -> (w48:T2)
      n15 = in-place-cluster #2("binary data"=w59) -> (w47:T2)
    }
    n16 = Replace Array Subset(array=w8, new element=w48, index=w49) -> (w45:T2[])
    n17 = Replace Array Subset(array=w45, new element=w47, index=w46) -> (w43:T2[])
    n18 = call <vilib>:"Generate Temporary File Path.vi"("error in (no error)"=w33, "Temporary File Extension (tmp)"="vi") -> ("error out"=w34:errorcluster, "Unique Temporary File Path"=w13:path)  [unwired: 8 in]
    n19 = call "Fix BDPW Checksum.vi"("Only fix 3rd hash (F)"=TRUE, "Resources"=w43) -> ("Resources out"=w42:T2[])  [unwired: 8 in, 1 out]
    n20 = call "Save Resource File.vi"("error in (no error)"=w34, "Path"=w13, "File type"="LVIN", "Resources"=w42) -> ("error out"=w18:errorcluster)  [unwired: 7 in]
    n21 = Open VI Reference(vi path=w13, error in (no error)=w18) -> (vi reference=w22:refnum<vi>, error out=w21:errorcluster)  [unwired: 4 in]
    n22 = call <vilib>:"Traverse for GObjects.vi"("Traverse Target"=TRef_TravTarget."FP", "error in (no error)"=w21, "Class Name"="Decoration", "VI Refnum"=w22) -> ("error out"=w12:errorcluster, "dup VI Refnum"=w14:refnum<vi>)  [unwired: 4 in, 2 out]
    "Last Error" <- w12
    n23 = Not(x=w12) -> (.not. x?=w23:bool)
    n24 = call <vilib>:"Clear Errors.vi"("error in (no error)"=w12) -> ("error out"=w15:errorcluster)  [unwired: 5 in, 1 out]
    n25 = case shown="True" w23 {
      tunnel: w25 -> [w55 w58]
      tunnel: w11 -> [_ w57]
      tunnel: [w55 w56] -> w24
      frame False {
      }
      frame True {
        n26 = Build Array (concatenate)(w58, w57) -> (w56:i32[])
      }
    }
    n27 = Close Reference(reference=w14, error in (no error)=w15) -> (error out=w16:errorcluster)
    n28 = Delete(path (use dialog)=w13, error in=w16) -> (error out=w17:errorcluster)  [unwired: 3 in, 2 out]
    "Working IDs" <- w25
    "i" <- w9
  }
  "error out" <- w4
